vi "Configure Burst.vi"(6 "Burst Count (1)":i32=1, 7 "Enable Burst (T: Enable)":bool=TRUE, 8 "error in (no error)":errorcluster, 9 "Burst Mode (0: Triggered)":u16(ring) items=["Triggered", "Gated"], 10 "Channel (1 Channel 1)":u16(ring)=1 items=["Channel 1"=1, "Channel 2"=2], 11 "VISA resource name":refnum<visa-resource-name>) -> (0 "error out":errorcluster, 3 "VISA resource name out":refnum<visa-resource-name>)   [LabVIEW 2016, in "Tektronix AFG 1000 Series.lvlib"]
doc: "Allows and configures burst modulation. Configures the function generator to output a waveform with specified number of cycles, called burst. The carrier waveform shape and parameters are set by Configure Standard Waveform."
uses:
  Tektronix AFG 1000 Series.lvlib
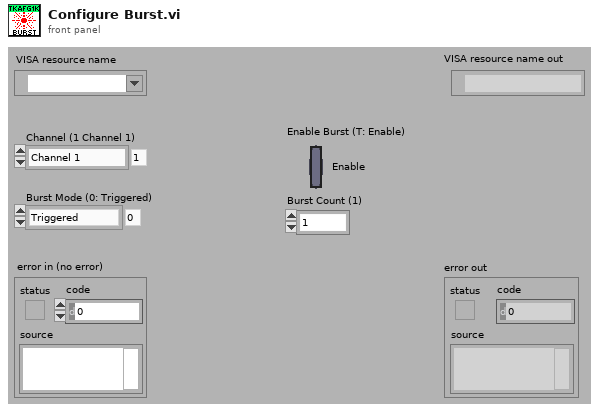
[diagram p1: front panel]
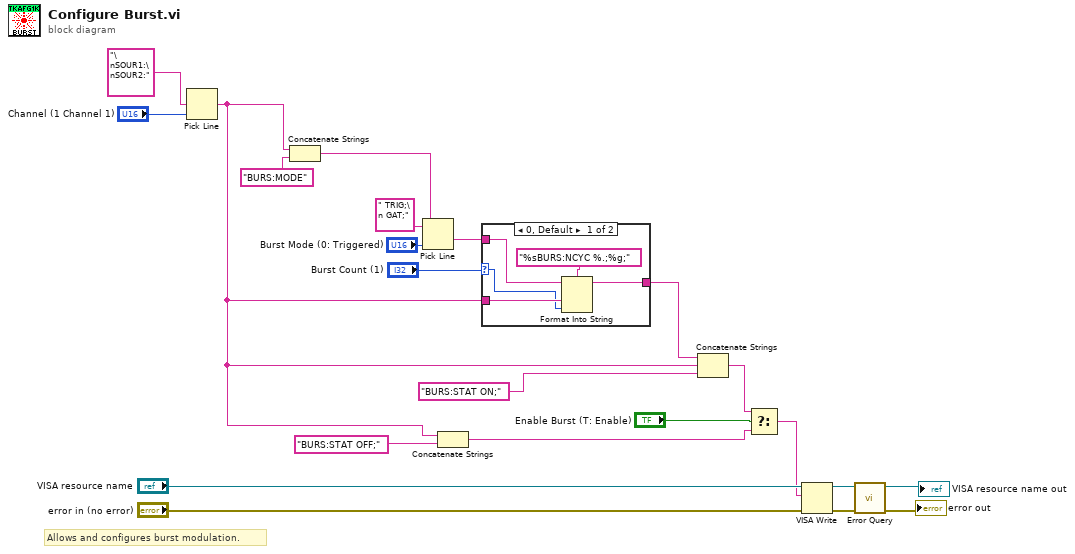
[diagram p0: block diagram]
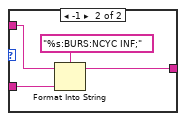
[diagram p2: hidden frame]
diagram:
  # "Allows and configures burst modulation."
  n1 = Pick Line(multi-line string="\nSOUR1:\nSOUR2:" ("string (\"\")"), line index="Channel (1 Channel 1)") -> (output string=w6:string)  [unwired: 1 in]
  n2 = Concatenate Strings(w6, "BURS:MODE" ("format string")) -> (w10:string)
  n3 = Pick Line(string ("")=w10, multi-line string=" TRIG;\n GAT;" ("string (\"\")"), line index="Burst Mode (0: Triggered)") -> (output string=w8:string)
  n4 = Concatenate Strings(w6, "BURS:STAT OFF;" ("string")) -> (w2:string)
  n5 = case shown="0, Default" "Burst Count (1)" {
    selector: "Burst Count (1)" -> [w23 _]
    tunnel: w6 -> [w27 w30]
    tunnel: w8 -> [w25 w29]
    tunnel: [w24 w28] -> w5
    frame 0, Default {
      n6 = Format Into String(format string="%sBURS:NCYC %.;%g;", initial string=w25, w27, w23) -> (resulting string=w24:string)  [unwired: 1 in, 1 out]
    }
    frame -1 {
      n7 = Format Into String(format string="%s:BURS:NCYC INF;", initial string=w29, w30) -> (resulting string=w28:string)  [unwired: 1 in, 1 out]
    }
  }
  n8 = Concatenate Strings(w5, w6, "BURS:STAT ON;" ("string")) -> (w4:string)
  n9 = Select(t=w4, s="Enable Burst (T: Enable)", f=w2) -> (s? t:f=w1:string)
  n10 = VISA Write(VISA resource name="VISA resource name", write buffer=w1, error in (no error)="error in (no error)") -> (VISA resource name out=w20:refnum<visa-resource-name>, error out=w19:errorcluster)  [unwired: 1 out]
  n11 = call "Error Query.vi"("error in (no error)"=w19, "VISA resource name"=w20) -> ("error out"=→"error out":errorcluster, "VISA resource name out"=→"VISA resource name out":refnum<visa-resource-name>)  [unwired: 6 in, 2 out]
